vi "Settings.vi"() -> ()   [LabVIEW 2013]
uses:
  TD GUI Settings.ctl
  qwtblvlib/TD Backend Engine.ctl
  qwtblvlib/TD Calculation Settings.ctl
  qwtblvlib/TD Uncertainty Calculation Method.ctl
  qwtblvlib/TD Correlation Calculation Settings.ctl
  qwtblvlib/TD DOF Calculation Settings.ctl
  qwtblvlib/TD MCM Calculation Settings.ctl
  qwtblvlib/TD MCM Calculation Method.ctl
  globals.vi
  <vilib>/Utility/xml.llb/Write to XML File(string).vi
  <vilib>/Utility/xml.llb/Read From XML File(string).vi
  qwtblvlib/QWTBLVLib.lvlib
panel:
  in  "hide this panel":bool
  out "Save data format":T9={"GUI Settings"={"Backend engine"=enum."Matlab by Script node", "QWTB Folder Path"=path ""}, "Calculation Settings"={"Strict"=FALSE, "Verbose"=TRUE, "Uncertainty Calculation Method"=enum."none", "Correlations"={"Required"=FALSE, "Generate"=FALSE}, "Degrees of Freedom"={"Required"=FALSE, "Generate"=FALSE}, "MCM Calculation Settings"={"Repeats"=100, "Verbose"=TRUE, "Parallelization method"=enum."Single Core", "Processors"=1, "Temporary directory"=".", "Randomize"=TRUE}}} {"Calculation Settings"."MCM Calculation Settings"."Processors" min=0 step=1; "Calculation Settings"."MCM Calculation Settings"."Repeats" min=1 step=1}
  in  "load":bool
  in  "save":bool
  in  "Calculation Settings":T3={"Strict"=TRUE, "Verbose"=TRUE, "Uncertainty Calculation Method"=enum."none", "Correlations"={"Required"=TRUE, "Generate"=TRUE}, "Degrees of Freedom"={"Required"=FALSE, "Generate"=TRUE}, "MCM Calculation Settings"={"Repeats"=100, "Verbose"=TRUE, "Parallelization method"=enum."Single Core", "Processors"=1, "Temporary directory"=".", "Randomize"=TRUE}} {"MCM Calculation Settings"."Processors" min=0 step=1; "MCM Calculation Settings"."Repeats" min=1 step=1}
  in  "GUI Settings":T1={"Backend engine"=enum."Matlab by Script node", "QWTB Folder Path"=path ""}
  # "Settings"
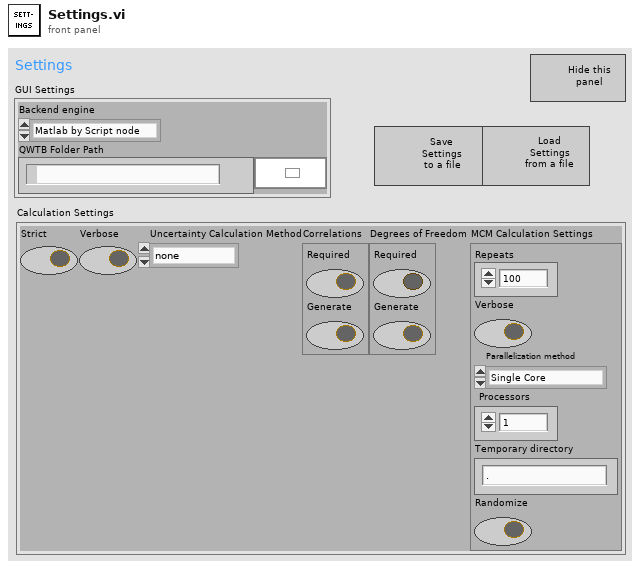
[diagram p1: front panel]
types:
  T1 = typedef "TD GUI Settings.ctl" = cluster{"Backend engine":T2, "QWTB Folder Path":path}
  T2 = typedef "QWTBLVLib.lvlib/TD Backend Engine.ctl" = enum16{"Matlab by Script node", "GNU Octave by GOLPI"}
  T3 = typedef "QWTBLVLib.lvlib/TD Calculation Settings.ctl" = cluster{"Strict":bool, "Verbose":bool, "Uncertainty Calculation Method":T4, "Correlations":T5, "Degrees of Freedom":T6, "MCM Calculation Settings":T7}
  T4 = typedef "QWTBLVLib.lvlib/TD Uncertainty Calculation Method.ctl" = enum16{"none", "GUF", "MCM"}
  T5 = typedef "QWTBLVLib.lvlib/TD Correlation Calculation Settings.ctl" = cluster{"Required":bool, "Generate":bool}
  T6 = typedef "QWTBLVLib.lvlib/TD DOF Calculation Settings.ctl" = cluster{"Required":bool, "Generate":bool}
  T7 = typedef "QWTBLVLib.lvlib/TD MCM Calculation Settings.ctl" = cluster{"Repeats":i32, "Verbose":bool, "Parallelization method":T8, "Processors":i32, "Temporary directory":string, "Randomize":bool}
  T8 = typedef "QWTBLVLib.lvlib/TD MCM Calculation Method.ctl" = enum16{"Single Core", "Multi Core", "Multi Station"}
  T9 = cluster{"GUI Settings":T1, "Calculation Settings":T3}
  T10 = enum32{"Invalid", "Standard", "Closed", "Hidden", "Minimized", "Maximized"}
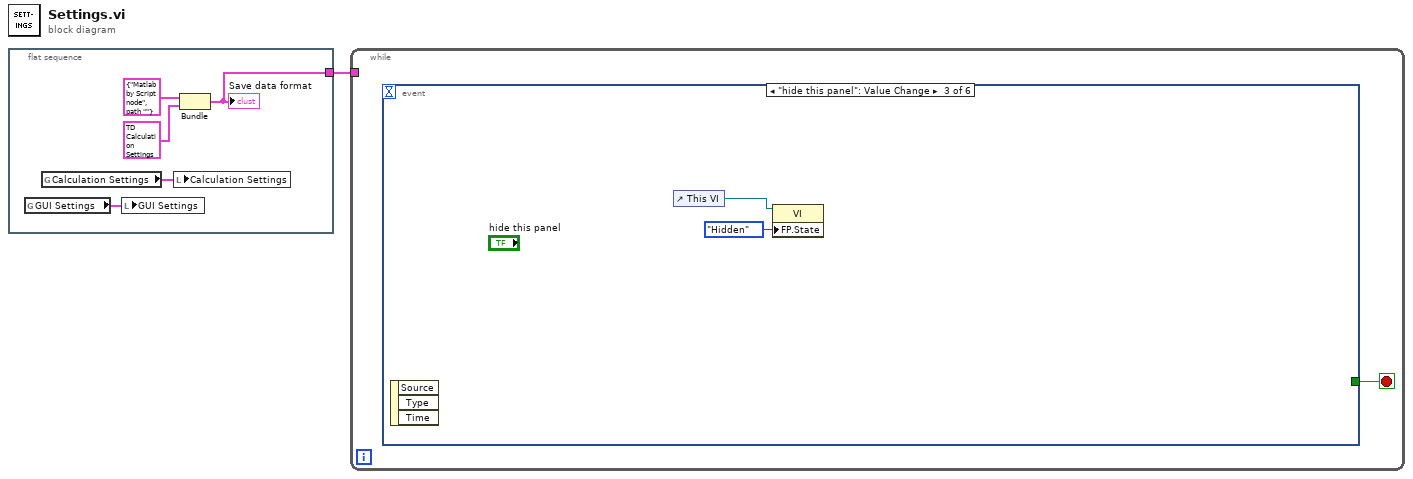
[diagram p0: block diagram]
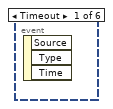
[diagram p2: hidden frame]
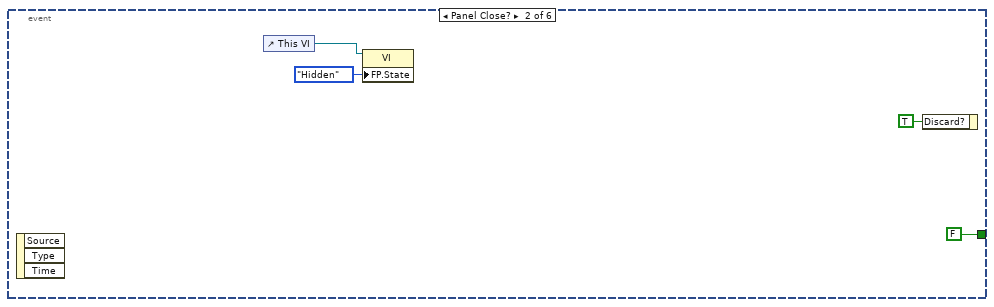
[diagram p3: hidden frame]
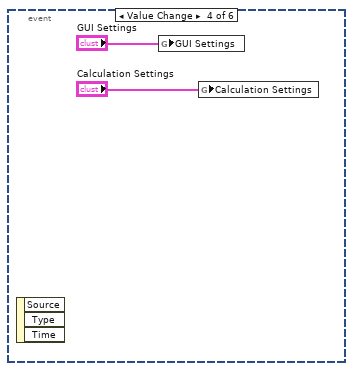
[diagram p4: hidden frame]
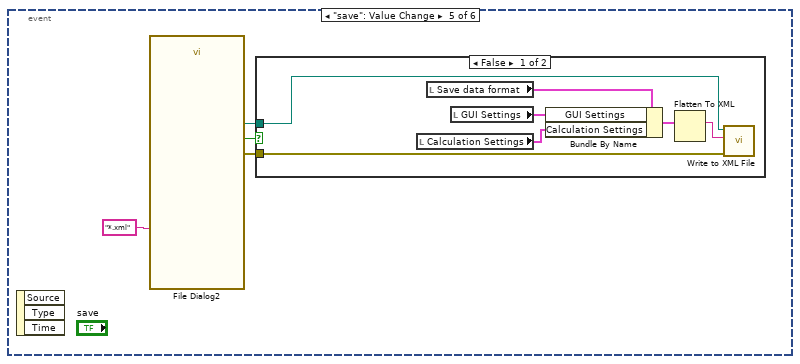
[diagram p5: hidden frame]
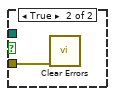
[diagram p6: hidden frame]
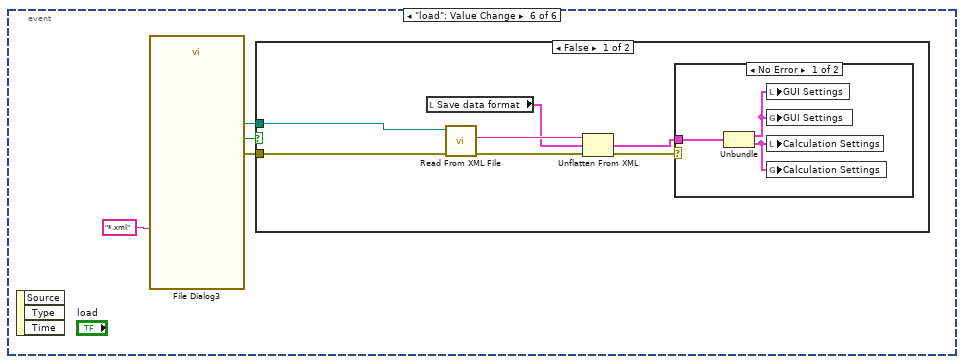
[diagram p7: hidden frame]
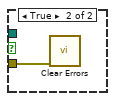
[diagram p9: hidden frame]
diagram:
  n1 = flat-sequence {
    tunnel: [w3] -> w1
    frame #0 {
      n2 = global read "globals.vi" "GUI Settings"() -> (w6:T1)
      n3 = global read "globals.vi" "Calculation Settings"() -> (w2:T3)
      n4 = local write "GUI Settings"(w6) -> ()
      n5 = local write "Calculation Settings"(w2) -> ()
      n6 = Bundle("GUI Settings"=T1 {"Backend engine"=enum."Matlab by Script node", "QWTB Folder Path"=path ""}, "Calculation Settings"=T3 {"Strict"=TRUE, "Verbose"=FALSE, "Uncertainty Calculation Method"=enum."none", "Correlations"={"Required"=TRUE, "Generate"=TRUE}, "Degrees of Freedom"={"Required"=FALSE, "Generate"=TRUE}, "MCM Calculation Settings"={"Repeats"=0, "Verbose"=FALSE, "Parallelization method"=enum."Single Core", "Processors"=0, "Temporary directory"="", "Randomize"=FALSE}}) -> (w3:T9)  [unwired: 1 in]
      "Save data format" <- w3
    }
  }
  n7 = while {
    tunnel: w1 -> [_]
    stop <- w7 stop-if-true
    n8 = event shown="[2] \"hide this panel\": Value Change" {
      selector: _ -> [_ _ _ _ _ _]
      dyn-events: _ -> [_ _ _ _ _ _]
      timeout: _ -> [_ _ _ _ _ _]
      tunnel: [_ FALSE ("cancel") _ _ _ _] -> w7
      event Timeout {
        n9 = event-data() -> ()  [unwired: 1 in, 3 out]
      }
      event Panel Close? {
        n10 = event-data() -> ()  [unwired: 1 in, 3 out]
        n11 = control-ref of="This VI"() -> (w9:refnum<vi>)
        n12 = property class="VI"(reference=w9, "FP.State"=T10."Hidden" ("Front Panel Window:State")) -> ()  [unwired: 1 in, 2 out]
        n13 = event-data("Discard?"=TRUE) -> ()  [unwired: 1 in, 1 out]
      }
      event "hide this panel": Value Change {
        n14 = event-data() -> ()  [unwired: 1 in, 3 out]
        n15 = control-ref of="This VI"() -> (w13:refnum<vi>)
        n16 = property class="VI"(reference=w13, "FP.State"=T10."Hidden" ("Front Panel Window:State")) -> ()  [unwired: 1 in, 2 out]
      }
      event Value Change {
        n17 = event-data() -> ()  [unwired: 1 in, 3 out]
        n18 = global write "globals.vi" "GUI Settings"("GUI Settings") -> ()
        n19 = global write "globals.vi" "Calculation Settings"("Calculation Settings") -> ()
      }
      event "save": Value Change {
        n20 = event-data() -> ()  [unwired: 1 in, 3 out]
        n21 = call "File Dialog2"("pattern (all files)"="*.xml") -> ("selected path"=w16:path, "cancelled"=w18:bool, "error out"=w17:errorcluster)  [unwired: 11 in, 1 out]
        n22 = case shown="False" w18 {
          tunnel: w17 -> [w25 w27]
          tunnel: w16 -> [w26 _]
          frame False {
            n23 = local read "Calculation Settings"() -> (w22:T3)
            n24 = local read "Save data format"() -> (w20:T9)
            n25 = local read "GUI Settings"() -> (w23:T1)
            n26 = Bundle By Name(cluster=w20, "GUI Settings"=w23, "Calculation Settings"=w22) -> (w21:T9)
            n27 = Flatten To XML(anything=w21) -> (xml string=w24:string)
            n28 = call-poly <vilib>:"Write to XML File.vi"("error in (no error)"=w25, "XML Input"=w24, "XML File Path"=w26) -> ()  [unwired: 6 in, 3 out]
          }
          frame True {
            n29 = call <vilib>:"Clear Errors.vi"("error in (no error)"=w27) -> ()  [unwired: 6 in, 1 out]
          }
        }
      }
      event "load": Value Change {
        n30 = event-data() -> ()  [unwired: 1 in, 3 out]
        n31 = call "File Dialog3"("pattern (all files)"="*.xml") -> ("selected path"=w28:path, "cancelled"=w30:bool, "error out"=w29:errorcluster)  [unwired: 11 in, 1 out]
        n32 = case shown="False" w30 {
          tunnel: w29 -> [w37 w42]
          tunnel: w28 -> [w38 _]
          frame False {
            n33 = local read "Save data format"() -> (w32:T9)
            n34 = call-poly <vilib>:"Read From XML File.vi"("error in (no error)"=w37, "XML File Path"=w38) -> ("error out"=w35:errorcluster, "XML Elements"=w36:string)  [unwired: 7 in, 1 out]
            n35 = Unflatten From XML(xml string=w36, type=w32, error in (no error)=w35) -> (value=w33:T9, error out=w34:errorcluster)
            n36 = case shown="No Error" w34 {
              tunnel: w33 -> [w41 _]
              frame No Error {
                n37 = Unbundle(w41) -> ("GUI Settings"=w40:T1, "Calculation Settings"=w39:T3)
                n38 = local write "GUI Settings"(w40) -> ()
                n39 = global write "globals.vi" "GUI Settings"(w40) -> ()
                n40 = local write "Calculation Settings"(w39) -> ()
                n41 = global write "globals.vi" "Calculation Settings"(w39) -> ()
              }
              frame Error {
              }
            }
          }
          frame True {
            n42 = call <vilib>:"Clear Errors.vi"("error in (no error)"=w42) -> ()  [unwired: 6 in, 1 out]
          }
        }
      }
    }
  }
